vi "Labspec Autofocus.vi"(8 "error in":errorcluster, 11 "Automation Refnum In":refnum<k7>) -> (0 "error out":errorcluster, 3 "Automation Refnum Out":refnum<k7>)   [LabVIEW 2014]
uses:
  Autofocus Mode.ctl
panel:
  out "Return":i32
  in  "Mode":T1 items=["Start"=0, "Status"=1, "Stop"=2, "Get Offset"=3, "Get State"=4, "Enable"=5, "Disable"=6, "Laser Autofocus"=10, "Raman Autofocus"=11, "Video Autofocus"=12]
  # "LICENSED MATERIALS – PROPERTY OF IBM\nCopyright IBM Corp. 2016, 2016\nALL RIGHTS RESERVED"
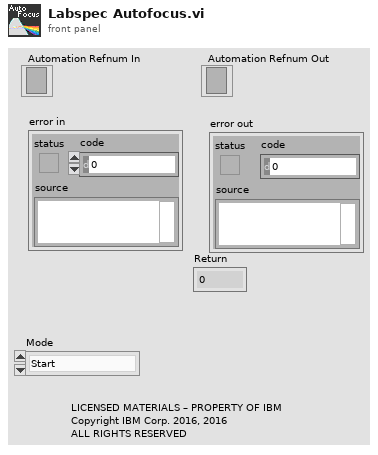
[diagram p1: front panel]
types:
  T1 = typedef "Autofocus Mode.ctl" = u16
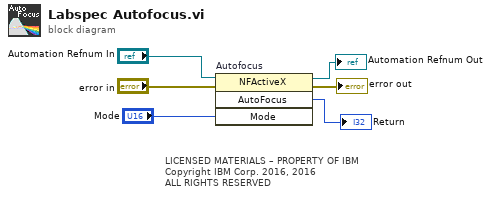
[diagram p0: block diagram]
diagram:
  # "LICENSED MATERIALS – PROPERTY OF IBM\nCopyright IBM Corp. 2016, 2016\nALL RIGHTS RESERVED"
  n1 = invoke on="Autofocus" class="NFActiveX" method="AutoFocus"(reference="Automation Refnum In", error in="error in", "Mode"="Mode") -> (reference out=→"Automation Refnum Out":refnum<k7>, error out=→"error out":errorcluster, "AutoFocus"=→"Return":i32)  [unwired: 1 in, 1 out]
